vi "Test_WriteItemTwice_DifferentTypes_Error.vi"(8 "error in (no error)":errorcluster, 11 "TestCase in":refnum<class "TestComposedLookupTable.lvclass">) -> (0 "error out":errorcluster, 3 "TestCase out":refnum<class "TestComposedLookupTable.lvclass">)   [LabVIEW 2017, in "TestComposedLookupTable.lvclass"]
uses:
  TestComposedLookupTable.lvclass
  Source/LookupTable/LookupTable.lvclass/LookupTable.ctl
  ff1124f4-1f02-4224-b17d-273dccbeca62.vi
  fe1e3695-476d-4265-a34a-e4fa04736bda.vi
  Source/LookupTable/Read Table Reference.vi
  ff1124f4-1f02-4224-b17d-273dccbeca62.vi/83a2748a-aded-4bad-b89d-cf0cdbc56d1f.vi
  fe1e3695-476d-4265-a34a-e4fa04736bda.vi/f16786c3-f291-4779-bd31-4112e4375cf4.vi
  Source/LookupTable/LookupTable.lvclass
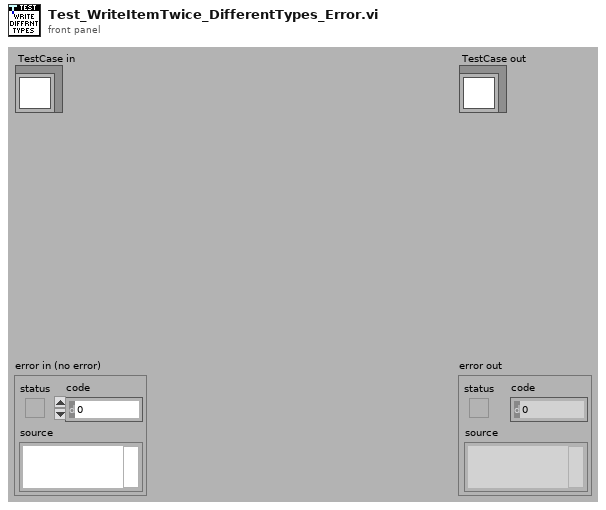
[diagram p1: front panel]
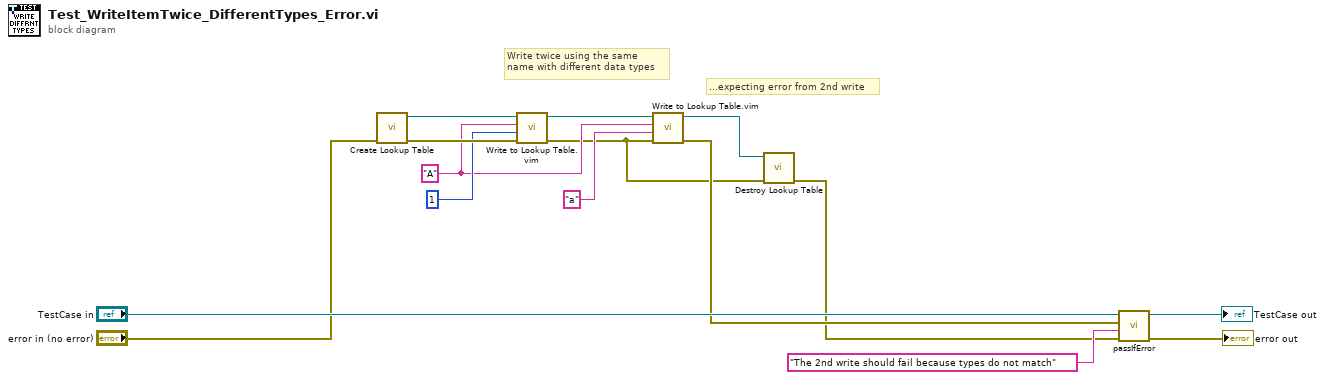
[diagram p0: block diagram]
diagram:
  w8 = "A" ("Item Name")
  # "...expecting error from 2nd write"
  # "Write twice using the same\nname with different data types"
  n1 = call "Create Lookup Table.vi"("error in (no error)"="error in (no error)") -> ("error out"=w15:errorcluster, "LookupTable Reference"=w1:refnum<data-value>)  [unwired: 9 in]
  n2 = call "Write to Lookup Table.vim"("error in (no error)"=w15, "Item"=1, "Item Name"=w8, "LookupTable Reference"=w1) -> ("error out"=w3:errorcluster, "LookupTable Reference Out"=w11:refnum<data-value>)  [unwired: 5 in, 1 out]
  n3 = call "Write to Lookup Table.vim"("error in (no error)"=w3, "Item"="a", "Item Name"=w8, "LookupTable Reference"=w11) -> ("error out"=w6:errorcluster, "LookupTable Reference Out"=w4:refnum<data-value>)  [unwired: 5 in, 1 out]
  n4 = call "Destroy Lookup Table.vi"("error in (no error)"=w3, "LookupTable Reference"=w4) -> ("error out"=w2:errorcluster)  [unwired: 9 in]
  n5 = call-dynamic "passIfError.vi"("error in (no error)"=w2, "task (\"\")"="The 2nd write should fail because types do not match" ("message (\"\")"), "error"=w6, "TestCase in"="TestCase in") -> ("error out"=→"error out":errorcluster, "TestCase out"=→"TestCase out":refnum<class "TestComposedLookupTable.lvclass">)  [unwired: 6 in]
